vi "Sensors.vi"() -> ()   [LabVIEW 2020]
uses:
  <vilib>/Rock Robotics/SystemInterfaces/i2clib/i2c_bus.ctl
  <vilib>/Rock Robotics/SystemInterfaces/AI/FPGA_AIChannel.ctl
  <vilib>/Rock Robotics/WPI/ThirdParty/Phoenix-LabVIEW/Pigeon IMU/CTRE_PigeonIMU_TareType.ctl
  Team Code/Robot Global Data.vi
  <vilib>/Rock Robotics/WPI/ThirdParty/Phoenix-LabVIEW/Motor Controller/Get/CTRE_Phoenix_MotorController_IntegratedSensorData_TalonFX.vi
  <vilib>/Rock Robotics/WPI/ThirdParty/Phoenix-LabVIEW/Motor Controller/Get/CTRE_Phoenix_MotorController_GetSelectedSensorData.vi
  <vilib>/Rock Robotics/WPI/ThirdParty/Phoenix-LabVIEW/Pigeon IMU/CTRE_PigeonIMU_GetYPR.vi
  <vilib>/Rock Robotics/WPI/ThirdParty/Phoenix-LabVIEW/CANCoder/Get/CTRE_Phoenix_CANcoder_GetSensorData.vi
panel:
  out "error out":errorcluster
  in  "colorThreshold":dbl=300.0
  in  "I2C Bus":T1=enum."I2C MXP"
  in  "Blue Calibration":cluster{"R":dbl, "G":dbl, "B":dbl}={"R"=0.175926, "G"=0.433962, "B"=0.386792}
  in  "Red Calibration":cluster{"R":dbl, "G":dbl, "B":dbl}={"R"=0.462185, "G"=0.38843, "B"=0.15126}
  in  "Yellow Calibration":cluster{"R":dbl, "G":dbl, "B":dbl}={"R"=0.361, "G"=0.524, "B"=0.113}
  in  "Hysteresis":dbl=0.15 format="%#_13g"
  in  "Voltage Threshold":dbl=0.7 format="%#_13g"
  out "Color":u32(colorbox)
  out "Measured Color":cluster{"R":dbl, "G":dbl, "B":dbl}
  out "LoopTime (ms)":u32
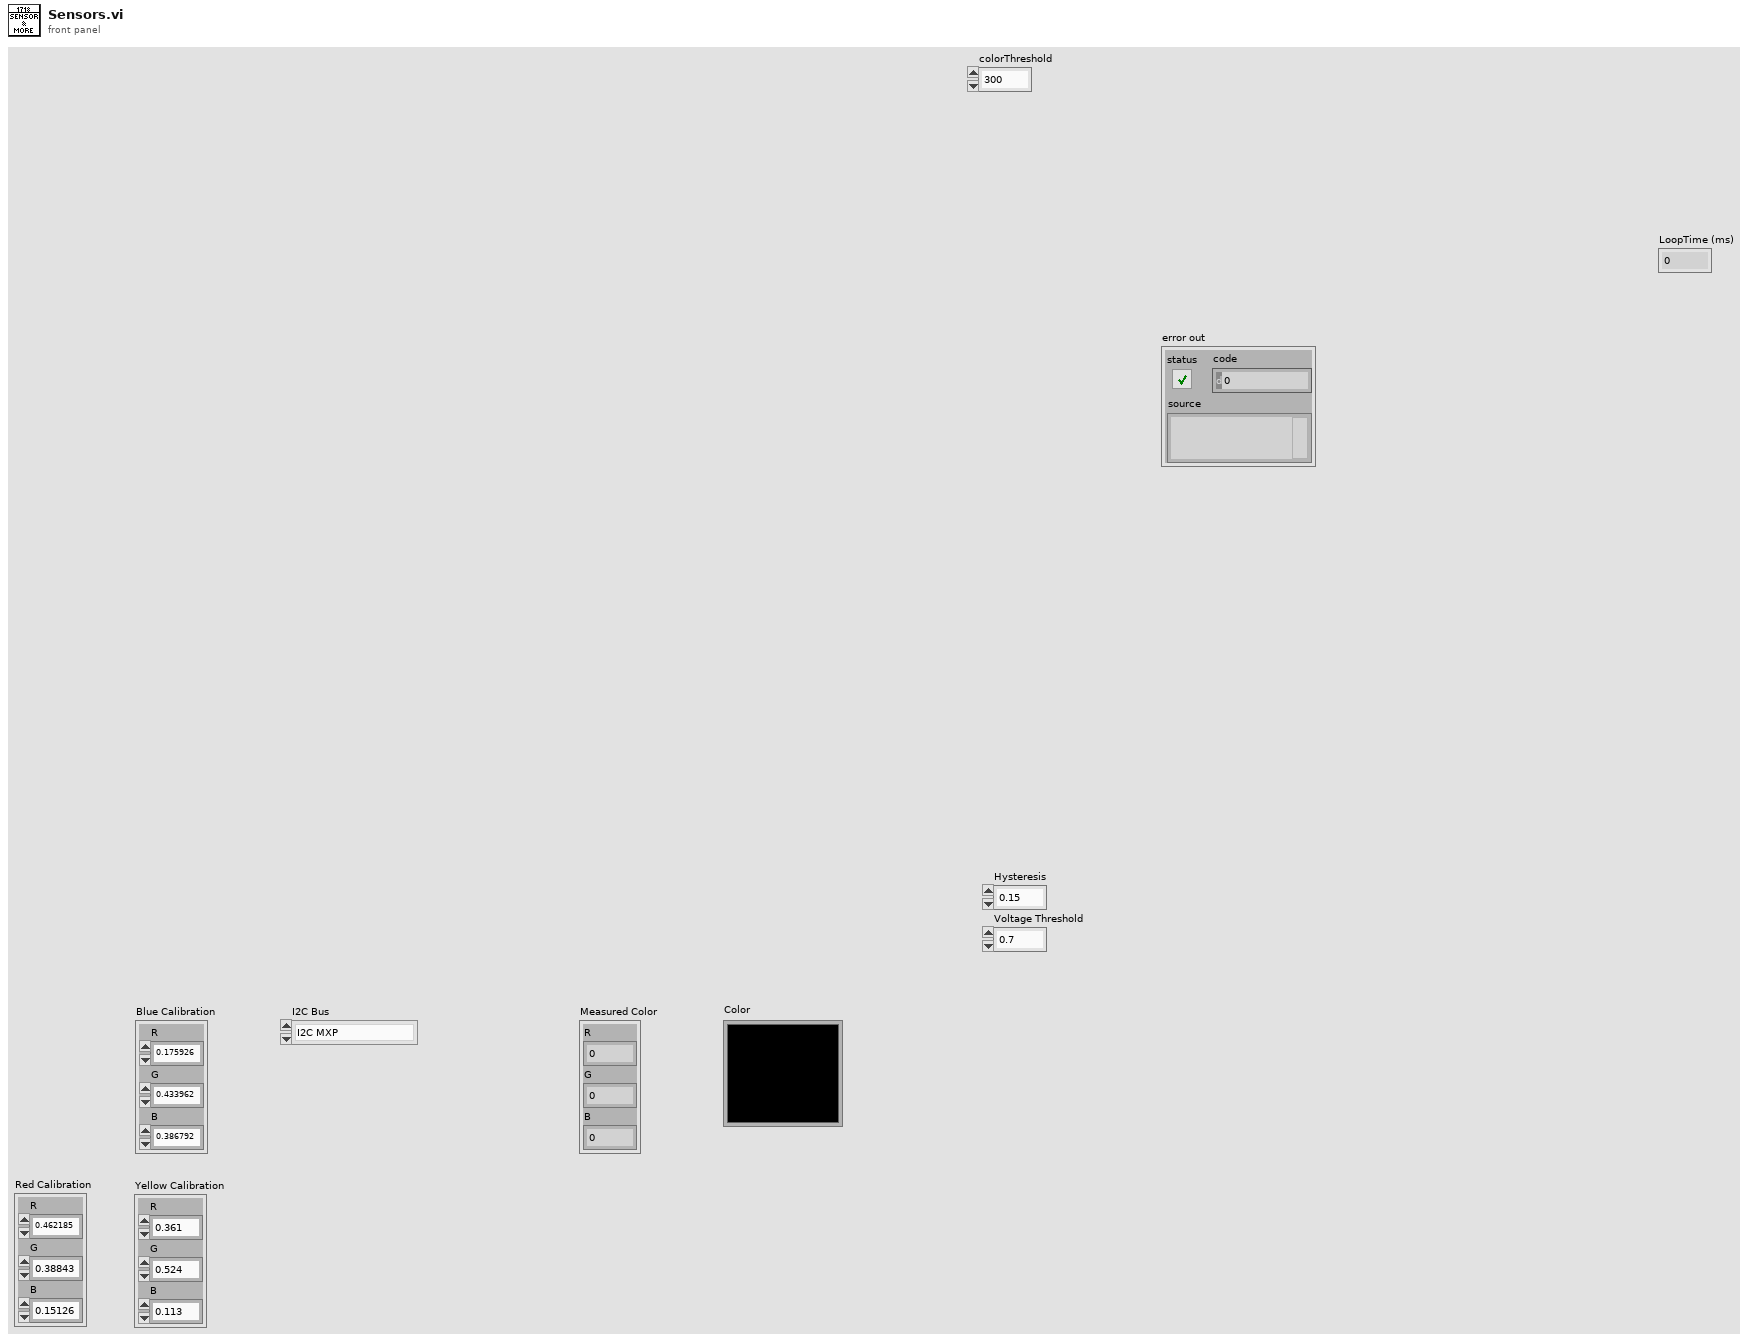
[diagram p1: front panel]
types:
  T1 = typedef "i2c_bus.ctl" = enum16{"I2C On-Board", "I2C MXP", "Invalid"}
  T2 = typedef "FPGA_AIChannel.ctl" = enum8{"AI 0", "AI 1", "AI 2", "AI 3", "AI MXP 0", "AI MXP 1", "AI MXP 2", "AI MXP 3", "Invalid"}
  T3 = typedef "PiConfig.ctl" = cluster{"swerveModules":cluster{"leftFront":T4, "rightFront":T4, "leftRear":T4, "rightRear":T4}, "offsets":cluster{"leftFrontAngleOffset":dbl, "leftRearAngleOffset":dbl, "rightFrontAngleOffset":dbl, "rightRearAngleOffset":dbl}, "limits":cluster{"maxVelocity":dbl, "maxOverdriveVelocity":dbl, "maxAcceleration":dbl, "maxPickupVelocity":dbl}, "speeds":cluster{"intakeSuckSpeed":dbl, "intakeSpitSpeed":dbl, "indexerSuckSpeed":dbl, "indexerSpitSpeed":dbl, "indexerShootSpeed":dbl, "indexerBumpBackSpeed":dbl, "shooterSpinupSpeed":dbl, "kickupSpinupSpeed":dbl, "shooterLowShootSpeed":dbl, "shooterHighShootSpeed":dbl}, "positions":cluster{"intakeStarting":dbl, "intakeStow":dbl, "intakeSuck":dbl, "armPounce":dbl, "armStow":dbl, "armUp":dbl, "winchPounce":dbl, "winchOut":dbl, "winchStow":dbl, "intakeSpit":dbl, "winchBarEngage":dbl, "winchBottomClimb":dbl, "hoodHighShoot":dbl, "armAirOut":dbl, "armAirUp":dbl, "winchAirOut":dbl, "winchAirUp":dbl, "winchHighClimb":dbl, "winchTraversalClimb":dbl}, "inversions":cluster{"rightShooter":bool, "leftShooter":bool}}
  T4 = typedef "Swerve Module Parameters.ctl" = cluster{"driveCANID":dbl, "angleCANID":i32, "canCoderCANID":dbl, "moduleName":string, "driveMotorNeutralMode":T5, "driveCurrentLimitConfig":T6, "driveFeedbackDevice":T7, "driveInitialSensorPosition":dbl, "driveEnableVoltageComp":bool, "driveVoltageComp":dbl, "driveRampRate":dbl, "angleCurrentLimit":dbl, "angleSensorType":T8, "angleMotorType":T9, "angleConversionFactor":dbl, "anglePIDRamp":dbl, "angleVoltageComp":dbl, "angleIdleMode":T10, "cancoderConfig":T11, "angleInitialSensorPosition":dbl}
  T5 = typedef "CTRE_Phoenix_MotorControl_NeutralMode.ctl" = enum8{"EEPROMSetting", "Override to Coast", "Override to Brake"}
  T6 = typedef "CTRE_Phoenix_MotorControl_SupplyCurrentLimitConfiguration.ctl" = cluster{"Enable?":bool, "Current Limit":dbl, "Threshold Current":dbl, "Threshold Time":dbl}
  T7 = typedef "CTRE_Phoenix_MotorControl_FeedbackDevice_TalonFX.ctl" = i8
  T8 = typedef "Spark MAX Sensor Type.ctl" = enum16{"No Sensor", "Hall Sensor", "Encoder", "-Not Available-", "Analog", "Alternate Encoder"}
  T9 = typedef "Spark MAX Motor Type.ctl" = enum16{"Brushed", "Brushless"}
  T10 = typedef "Spark MAX Idle Mode.ctl" = enum16{"Coast", "Brake"}
  T11 = typedef "CTRE_Phoenix_CANcoder_Configurables.ctl" = cluster{"Sensor Initialization Strategy":T12, "Absolute Sensor Range":T13, "Velocity Measurement Period":T14, "Velocity Measurement Window":i32, "Magnet Offset (Degrees)":dbl, "Sensor Direction":bool, "Sensor Coefficient":dbl, "Unit String":string, "Sensor Time Base":T15}
  T12 = typedef "CTRE_Phoenix_CANcoder_SensorInitializationStrategy.ctl" = enum16{"Boot To Zero", "Boot To Absolute Position"}
  T13 = typedef "CTRE_Phoenix_CANcoder_AbsoluteSensorRange.ctl" = enum16{"Unsigned [0 to 360)", "Signed [-180 to +180)"}
  T14 = typedef "CTRE_Phoenix_MotorControl_VelocityMeasurementPeriod.ctl" = u16
  T15 = typedef "CTRE_Phoenix_CANcoder_SensorTimeBase.ctl" = enum16{"Per100Ms_Legacy", "PerSecond", "PerMinute"}
  T16 = typedef "Color Sensor V3 DevRef.ctl" = cluster{"I2CDevRef":T17}
  T17 = typedef "WPI_I2CDevRef.ctl" = cluster{"DevStatus":errorcluster, "Device Address":u8, "Handle":i32, "I2C Bus":T1}
  T18 = typedef "WPI_AnalogChannelDevRef.ctl" = cluster{"DevStatus":errorcluster, "Analog Channel":T2}
  T19 = typedef "CTRE_Phoenix_CANcoder_DeviceRef.ctl" = cluster{"DeviceStatus":errorcluster, "Device Number":u8, "Handle":u64, "UsageFrame":u32, "Library Path":path}
  T20 = typedef "WPI_MotorControlDeviceRef.ctl" = cluster{"DeviceStatus":errorcluster, "Type":T21, "PWM":cluster{"PWM Channel":T22, "DeadBand":T23}, "CAN":cluster{"Device Number":u8, "SetOutput VI Ref":variant, "GetOutput VI Ref":variant, "Enable VI Ref":variant, "Disable VI Ref":variant, "Data":variant}, "Invert":bool, "DIO PWM":cluster{"PWM \"Enable\" Channel":T22, "DIOChannel":T24, "PWM Rate":dbl}}
  T21 = typedef "WPI_MotorControlType.ctl" = enum16{"PWM", "CAN", "DIO PWM"}
  T22 = typedef "FPGA_DIOPWMChannel.ctl" = enum8{"PWM 0", "PWM 1", "PWM 2", "PWM 3", "PWM 4", "PWM 5", "PWM 6", "PWM 7", "PWM 8", "PWM 9", "PWM MXP 0", "PWM MXP 1", "PWM MXP 2", "PWM MXP 3", "PWM MXP 4", "PWM MXP 5", "PWM MXP 6", "PWM MXP 7", "PWM MXP 8", "PWM MXP 9", "Invalid"}
  T23 = typedef "WPI_PWMDeadband.ctl" = cluster{"Name":string, "maxPositivePwm":i32, "minPositivePwm":i32, "centerPwm":i32, "maxNegativePwm":i32, "minNegativePwm":i32, "angularRange":u16}
  T24 = typedef "FPGA_DIOChannel.ctl" = enum8{"DIO 0", "DIO 1", "DIO 2", "DIO 3", "DIO 4", "DIO 5", "DIO 6", "DIO 7", "DIO 8", "DIO 9", "DIO MXP 0", "DIO MXP 1", "DIO MXP 2", "DIO MXP 3", "DIO MXP 4", "DIO MXP 5", "DIO MXP 6", "DIO MXP 7", "DIO MXP 8", "DIO MXP 9", "DIO MXP 10", "DIO MXP 11", "DIO MXP 12", "DIO MXP 13", "DIO MXP 14", "DIO MXP 15", "SPI Port CS1", "SPI Port CS2", "SPI Port CS3", "SPI Port MISO", "SPI Port MOSI", "Invalid"}
  T25 = typedef "CTRE_PigeonIMU_DeviceRef.ctl" = cluster{"DeviceStatus":errorcluster, "Device Number":u8, "Type":T26, "Device ID":u32, "Handle":u64, "UsageFrame":u32, "Library Path":path}
  T26 = typedef "CTRE_PigeonIMU_ConnectionType.ctl" = u32
  T27 = typedef "WPI_DriverStationAllianceInfo.ctl" = enum16{"Red", "Blue", "Invalid"}
  T28 = typedef "CTRE_PigeonIMU_TareType.ctl" = u8
  T29 = cluster{"offsetAngle H":dbl, "offsetAngle V":dbl, "area":dbl, "skew":dbl}
  T30 = cluster{"rightFrontDrivePositionTicks":dbl, "leftFrontDrivePositionTicks":dbl, "leftRearDrivePositionTicks":dbl, "rightRearDrivePositionTicks":dbl}
  T31 = cluster{"leftFrontDriveVelocityTicksPer100ms":dbl, "leftRearDriveVelocityTicksPer100ms":dbl, "rightFrontDriveVelocityTicksPer100ms":dbl, "rightRearDriveVelocityTicksper100ms":dbl}
  T32 = typedef "Absolute Angle TypeDef.ctl" = cluster{"leftFrontAbsoluteAngle":dbl, "leftRearAbsoluteAngle":dbl, "rightFrontAbsoluteAngle":dbl, "rightRearAbsoluteAngle":dbl}
  T33 = typedef "Cargo Sensors.ctl" = cluster{"ballPresent0":bool, "ballPresent1":bool, "ballPresent2":bool, "colorIsCorrect":bool, "ballPresent3":bool}
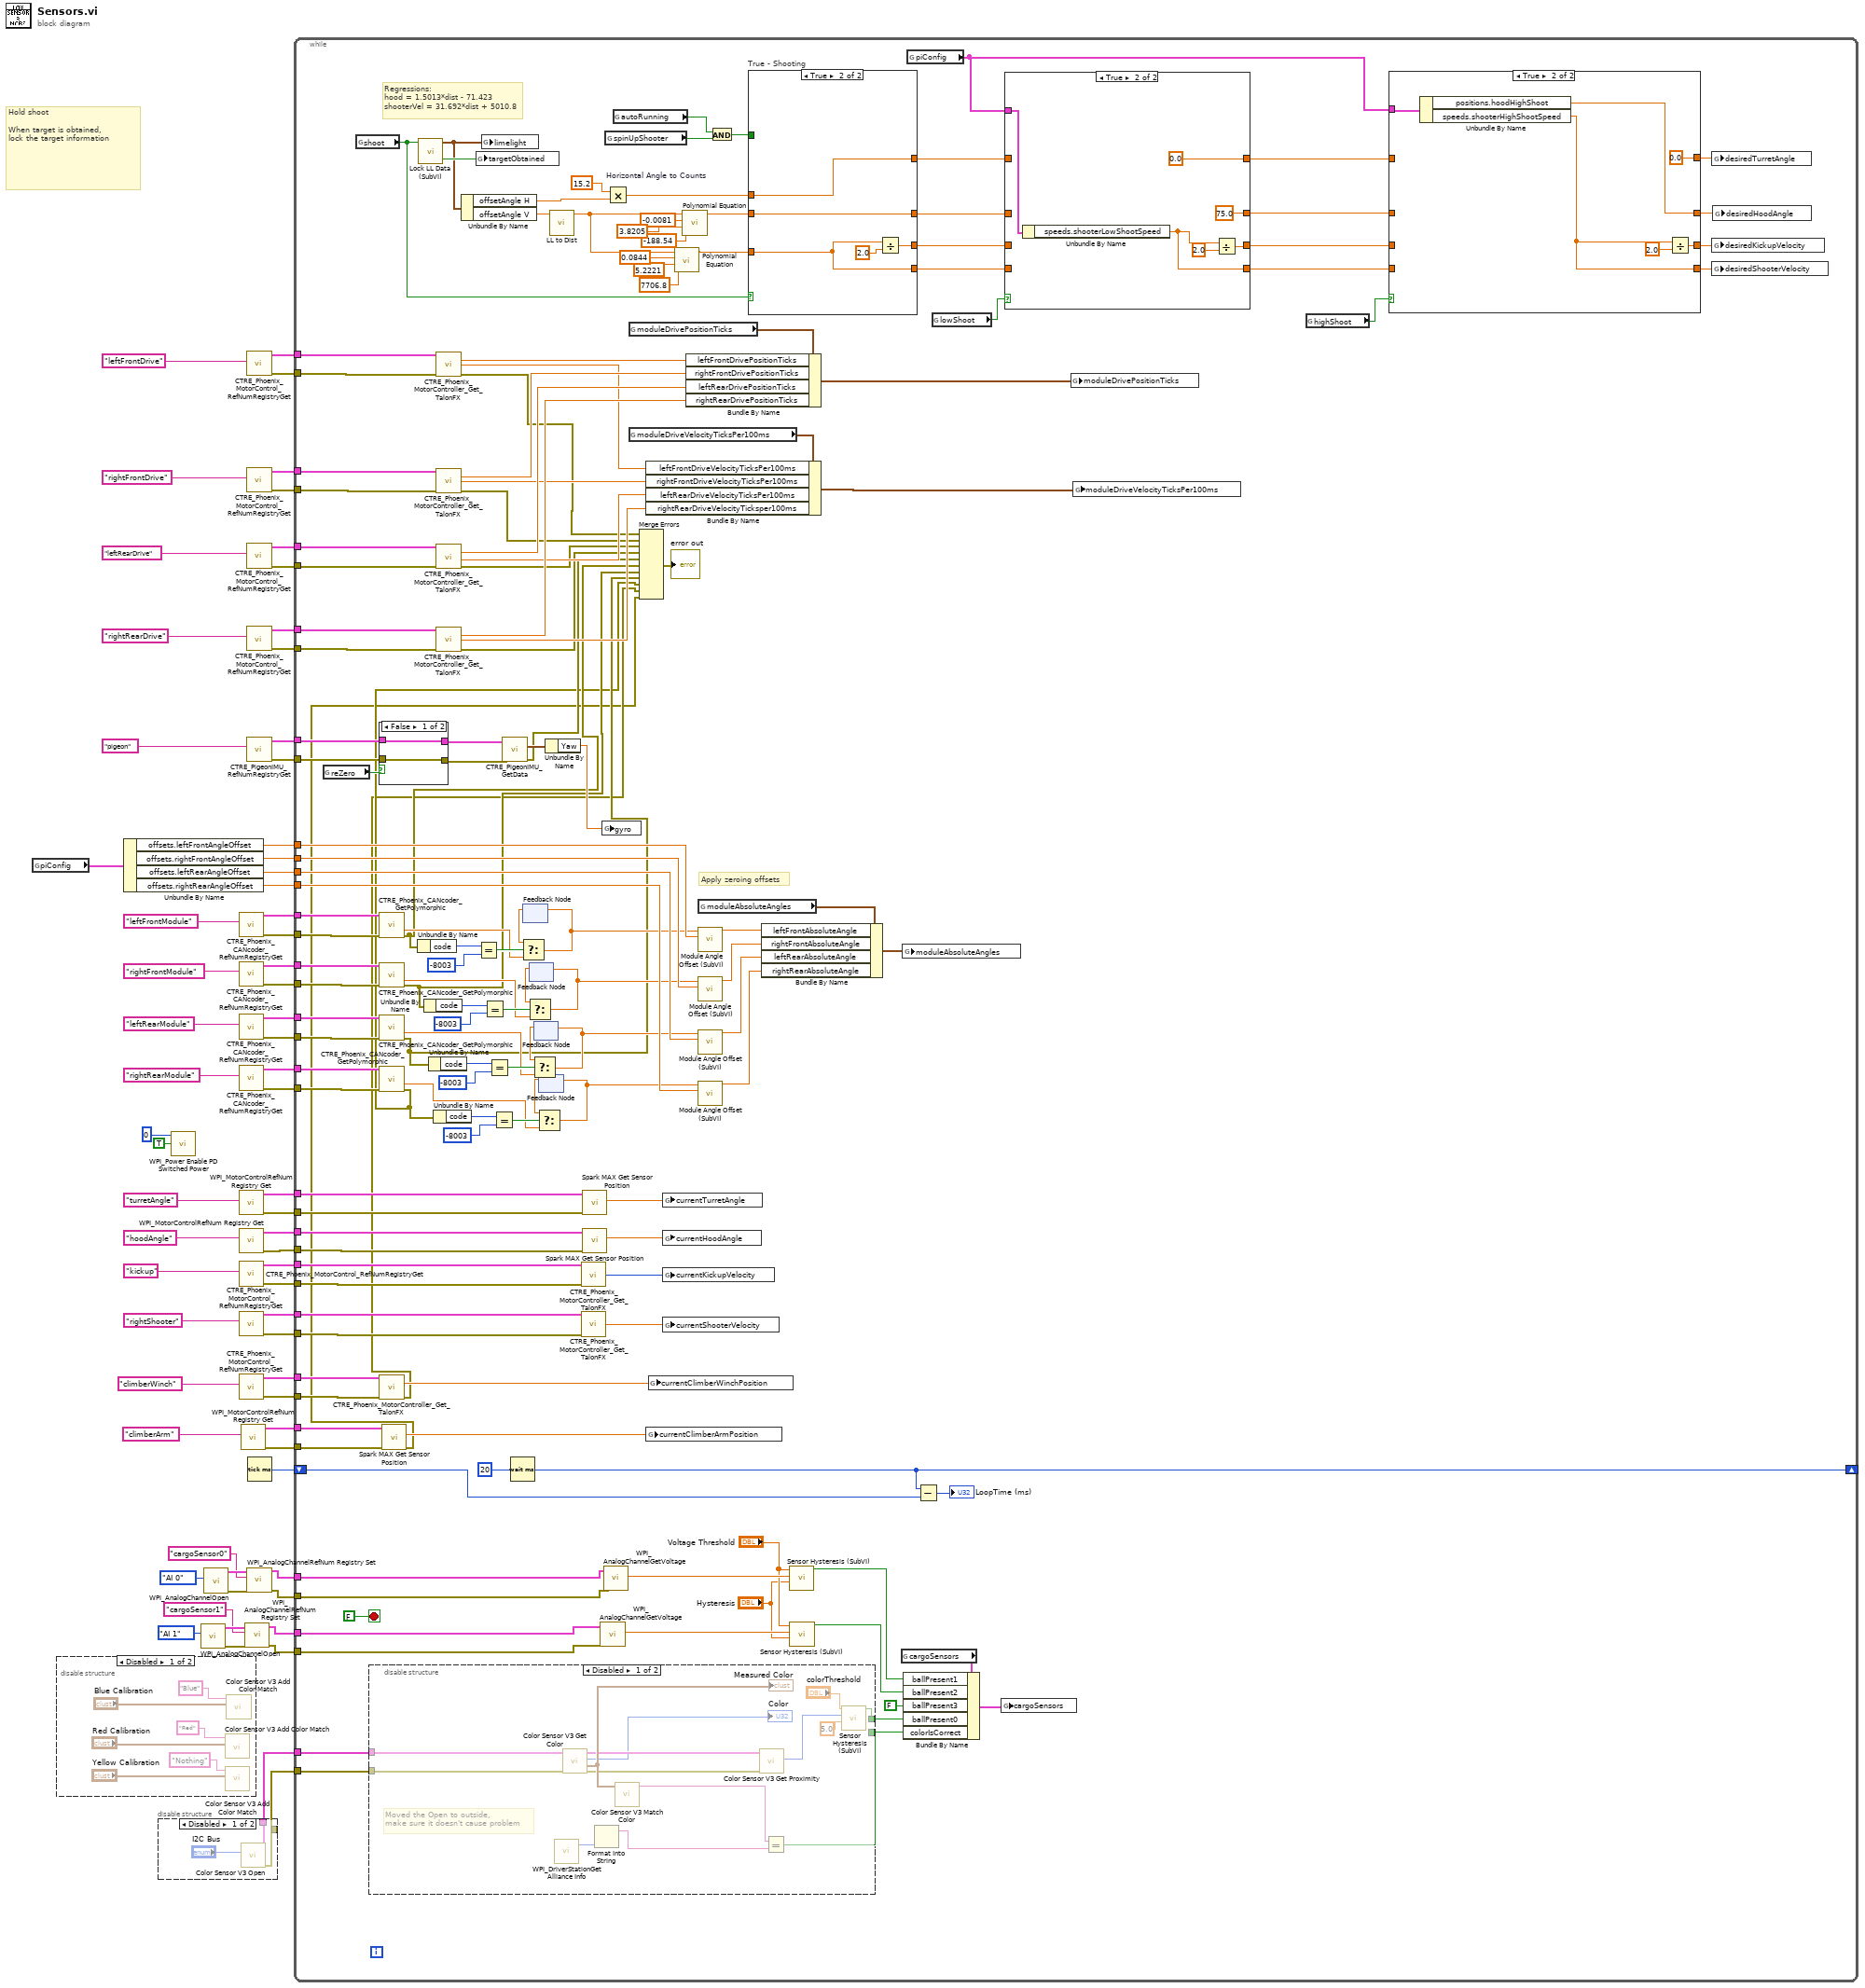
[diagram p0: block diagram]
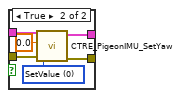
[diagram p4: hidden frame]
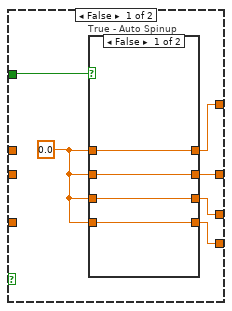
[diagram p8: hidden frame]
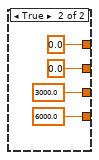
[diagram p9: hidden frame]
diagram:
  # "Hold shoot\n\nWhen target is obtained,\nlock the target information"
  n1 = global read "Robot Global Data.vi" "piConfig"() -> (w55:T3)
  n2 = disable-structure shown="Disabled" {
    frame Disabled {
      n3 = call <vilib>:"Color Sensor V3 Add Color Match.vi"("Color"="Red Calibration", "Name"="Red") -> ()  [unwired: 10 in]
      n4 = call <vilib>:"Color Sensor V3 Add Color Match.vi"("Color"="Yellow Calibration", "Name"="Nothing") -> ()  [unwired: 10 in]
      n5 = call <vilib>:"Color Sensor V3 Add Color Match.vi"("Color"="Blue Calibration", "Name"="Blue") -> ()  [unwired: 10 in]
    }
    frame Enabled {
    }
  }
  n6 = Unbundle By Name(w55) -> ("offsets.leftFrontAngleOffset"=w49:dbl, "offsets.rightFrontAngleOffset"=w48:dbl, "offsets.leftRearAngleOffset"=w47:dbl, "offsets.rightRearAngleOffset"=w46:dbl)
  n7 = disable-structure shown="Disabled" {
    disable-tunnel: [w76 _] -> w18
    disable-tunnel: [w75 _] -> w17
    frame Disabled {
      n8 = call <vilib>:"Color Sensor V3 Open.vi"("I2C Bus"="I2C Bus") -> ("error out"=w76:errorcluster, "ColorSensorDevRef"=w75:T16)  [unwired: 9 in]
    }
    frame Enabled {
    }
  }
  n9 = call <vilib>:"WPI_Power Enable PD Switched Power.vi"("Power Distribution (def)"=u8 0, "Switch Channel Value"=TRUE) -> ()  [unwired: 12 in, 2 out]
  n10 = call <vilib>:"WPI_AnalogChannelOpen.vi"("Analog Channel"=FPGA_AIChannel."AI 1") -> ("error out"=w16:errorcluster, "AIDeviceRef"=w15:T18)  [unwired: 9 in]
  n11 = call <vilib>:"WPI_AnalogChannelOpen.vi"("Analog Channel"=FPGA_AIChannel."AI 0") -> ("error out"=w13:errorcluster, "AIDeviceRef"=w14:T18)  [unwired: 9 in]
  n12 = call <vilib>:"CTRE_Phoenix_CANcoder_RefNumRegistryGet.vi"("refnum name"="leftFrontModule") -> ("error out"=w44:errorcluster, "CTRE_CANcoder_DeviceRef"=w45:T19)  [unwired: 9 in]
  n13 = call <vilib>:"CTRE_Phoenix_CANcoder_RefNumRegistryGet.vi"("refnum name"="rightFrontModule") -> ("error out"=w42:errorcluster, "CTRE_CANcoder_DeviceRef"=w43:T19)  [unwired: 9 in]
  n14 = call <vilib>:"CTRE_Phoenix_CANcoder_RefNumRegistryGet.vi"("refnum name"="leftRearModule") -> ("error out"=w40:errorcluster, "CTRE_CANcoder_DeviceRef"=w41:T19)  [unwired: 9 in]
  n15 = call <vilib>:"CTRE_Phoenix_CANcoder_RefNumRegistryGet.vi"("refnum name"="rightRearModule") -> ("error out"=w38:errorcluster, "CTRE_CANcoder_DeviceRef"=w39:T19)  [unwired: 9 in]
  n16 = call <vilib>:"WPI_MotorControlRefNum Registry Get.vi"("refnum name"="turretAngle") -> ("error out"=w32:errorcluster, "MotorControlDevRef"=w33:T20)  [unwired: 9 in]
  n17 = call <vilib>:"WPI_MotorControlRefNum Registry Get.vi"("refnum name"="hoodAngle") -> ("error out"=w31:errorcluster, "MotorControlDevRef"=w30:T20)  [unwired: 9 in]
  n18 = call <vilib>:"CTRE_Phoenix_MotorControl_RefNumRegistryGet.vi"("refnum name"="kickup") -> ("error out"=w25:errorcluster, "PhoenixMotorControlDevRef"=w26:T20)  [unwired: 9 in]
  n19 = call <vilib>:"CTRE_Phoenix_MotorControl_RefNumRegistryGet.vi"("refnum name"="rightShooter") -> ("error out"=w23:errorcluster, "PhoenixMotorControlDevRef"=w24:T20)  [unwired: 9 in]
  n20 = call <vilib>:"CTRE_Phoenix_MotorControl_RefNumRegistryGet.vi"("refnum name"="climberWinch") -> ("error out"=w8:errorcluster, "PhoenixMotorControlDevRef"=w7:T20)  [unwired: 9 in]
  n21 = call <vilib>:"WPI_MotorControlRefNum Registry Get.vi"("refnum name"="climberArm") -> ("error out"=w5:errorcluster, "MotorControlDevRef"=w4:T20)  [unwired: 9 in]
  n22 = call <vilib>:"WPI_AnalogChannelRefNum Registry Set.vi"("error in (no error)"=w16, "refnum name"="cargoSensor1", "AIDeviceRef"=w15) -> ("error out"=w22:errorcluster, "AIDeviceRef"=w21:T18)  [unwired: 7 in]
  n23 = call <vilib>:"CTRE_Phoenix_MotorControl_RefNumRegistryGet.vi"("refnum name"="leftFrontDrive") -> ("error out"=w62:errorcluster, "PhoenixMotorControlDevRef"=w63:T20)  [unwired: 9 in]
  n24 = call <vilib>:"CTRE_Phoenix_MotorControl_RefNumRegistryGet.vi"("refnum name"="rightFrontDrive") -> ("error out"=w60:errorcluster, "PhoenixMotorControlDevRef"=w61:T20)  [unwired: 9 in]
  n25 = call <vilib>:"CTRE_Phoenix_MotorControl_RefNumRegistryGet.vi"("refnum name"="leftRearDrive") -> ("error out"=w56:errorcluster, "PhoenixMotorControlDevRef"=w57:T20)  [unwired: 9 in]
  n26 = call <vilib>:"CTRE_Phoenix_MotorControl_RefNumRegistryGet.vi"("refnum name"="rightRearDrive") -> ("error out"=w58:errorcluster, "PhoenixMotorControlDevRef"=w59:T20)  [unwired: 9 in]
  n27 = call <vilib>:"CTRE_PigeonIMU_RefNumRegistryGet.vi"("refnum name"="pigeon") -> ("error out"=w36:errorcluster, "PigeonIMUDevRef"=w37:T25)  [unwired: 9 in]
  n28 = call <vilib>:"WPI_AnalogChannelRefNum Registry Set.vi"("error in (no error)"=w13, "refnum name"="cargoSensor0", "AIDeviceRef"=w14) -> ("error out"=w20:errorcluster, "AIDeviceRef"=w19:T18)  [unwired: 7 in]
  n29 = Tick Count (ms)() -> (millisecond timer value=w35:u32)
  n30 = while {
    tunnel: w63 -> [w231]
    tunnel: w62 -> [w230]
    tunnel: w61 -> [w229]
    tunnel: w60 -> [w228]
    tunnel: w59 -> [w227]
    tunnel: w58 -> [w226]
    tunnel: w57 -> [w225]
    tunnel: w56 -> [w224]
    tunnel: w49 -> [w222]
    tunnel: w48 -> [w221]
    tunnel: w47 -> [w220]
    tunnel: w46 -> [w219]
    tunnel: w45 -> [w218]
    tunnel: w44 -> [w217]
    tunnel: w43 -> [w216]
    tunnel: w42 -> [w215]
    tunnel: w41 -> [w214]
    tunnel: w40 -> [w213]
    tunnel: w39 -> [w212]
    tunnel: w38 -> [w211]
    tunnel: w37 -> [w103]
    tunnel: w36 -> [w102]
    shift-right: [w189] -> _
    shift-left: w35 -> [w190]
    tunnel: w33 -> [w187]
    tunnel: w32 -> [w188]
    tunnel: w30 -> [w186]
    tunnel: w31 -> [w185]
    tunnel: w26 -> [w182]
    tunnel: w25 -> [w181]
    tunnel: w24 -> [w180]
    tunnel: w23 -> [w179]
    tunnel: w22 -> [w173]
    tunnel: w21 -> [w172]
    tunnel: w20 -> [w171]
    tunnel: w19 -> [w170]
    tunnel: w18 -> [w163]
    tunnel: w17 -> [w162]
    tunnel: w7 -> [w124]
    tunnel: w8 -> [w125]
    tunnel: w4 -> [w121]
    tunnel: w5 -> [w120]
    stop <- FALSE stop-if-true
    # "Regressions:\nhood = 1.5013*dist - 71.423\nshooterVel = 31.692*dist + 5010.8"
    # "Apply zeroing offsets"
    n31 = global read "Robot Global Data.vi" "reZero"() -> (w99:bool)
    n32 = global read "Robot Global Data.vi" "shoot"() -> (w156:bool)
    n33 = disable-structure shown="Disabled" {
      disable-tunnel: [w273 _] -> w167
      disable-tunnel: [w272 _] -> w164
      disable-tunnel: w163 -> [w271 _]
      disable-tunnel: w162 -> [w270 _]
      frame Disabled {
        # "Moved the Open to outside,\nmake sure it doesn't cause problem"
        n34 = call <vilib>:"WPI_DriverStationGet Alliance Info.vi"() -> ("Alliance"=w268:T27)  [unwired: 6 in, 5 out]
        n35 = call <vilib>:"Color Sensor V3 Get Color.vi"("error in (no error)"=w271, "ColorSensorDevRef"=w270) -> ("error out"=w264:errorcluster, "Normalized Color"=w266:cluster{"R":dbl, "G":dbl, "B":dbl}, "Color"=→"Color":u32, "ColorSensorDevRef out"=w265:T16)  [unwired: 6 in]
        "Measured Color" <- w266
        n36 = Format Into String(w268) -> (resulting string=w269:string)  [unwired: 3 in, 1 out]
        n37 = call <vilib>:"Color Sensor V3 Match Color.vi"("Measured Color"=w266) -> ("Matched Color Name"=w267:string)  [unwired: 8 in, 2 out]
        n38 = call <vilib>:"Color Sensor V3 Get Proximity.vi"("error in (no error)"=w264, "ColorSensorDevRef"=w265) -> ("Proximity"=w261:u16)  [unwired: 7 in, 2 out]
        n39 = Equal?(x=w267, y=w269) -> (x = y?=w273:bool)
        n40 = call "Sensor Hysteresis (SubVI).vi"("Hysteresis"=5.0, "Input"=w261, "Threshold"="colorThreshold") -> ("Above Threshold"=w272:bool)  [unwired: 8 in]
      }
      frame Enabled {
      }
    }
    n41 = case shown="False" w99 {
      tunnel: w103 -> [w233 w239]
      tunnel: w102 -> [w232 w238]
      tunnel: [w233 w237] -> w101
      tunnel: [w232 w236] -> w100
      frame False {
      }
      frame True {
        w234 = T28 0 items=["SetValue"=0, "AddOffset"=1, "MatchCompass"=2, "SetOffset"=255] ("TareType (SetValue)")
        n42 = call <vilib>:"CTRE_PigeonIMU_SetYaw.vi"("error in (no error)"=w238, "TareType (SetValue)"=w234, "Value"=0.0, "PigeonIMUDevRef"=w239) -> ("error out"=w236:errorcluster, "PigeonIMUDevRef"=w237:T25)  [unwired: 6 in]
      }
    }
    n43 = call-poly <vilib>:"CTRE_Phoenix_CANcoder_GetPolymorphic.vi"("CTRE_CANcoder_DeviceRef"=w218, "error in"=w217) -> ("Absolute Position"=w145:dbl, "error out"=w83:errorcluster)  [unwired: 9 in, 3 out]
    n44 = call-poly <vilib>:"CTRE_Phoenix_CANcoder_GetPolymorphic.vi"("CTRE_CANcoder_DeviceRef"=w216, "error in"=w215) -> ("Absolute Position"=w131:dbl, "error out"=w82:errorcluster)  [unwired: 9 in, 3 out]
    n45 = call-poly <vilib>:"CTRE_Phoenix_CANcoder_GetPolymorphic.vi"("CTRE_CANcoder_DeviceRef"=w214, "error in"=w213) -> ("Absolute Position"=w129:dbl, "error out"=w81:errorcluster)  [unwired: 9 in, 3 out]
    n46 = call-poly <vilib>:"CTRE_Phoenix_CANcoder_GetPolymorphic.vi"("CTRE_CANcoder_DeviceRef"=w212, "error in"=w211) -> ("Absolute Position"=w128:dbl, "error out"=w80:errorcluster)  [unwired: 9 in, 3 out]
    n47 = call-poly <vilib>:"CTRE_Phoenix_MotorController_Get_TalonFX.vi"("PhoenixMotorControlDevRef"=w124, "error in"=w125) -> ("Position"=w123:dbl, "error out"=w79:errorcluster)  [unwired: 9 in, 3 out]
    n48 = call <vilib>:"Spark MAX Get Sensor Position.vi"("error in (no error)"=w120, "MotorControlDevRef in"=w121) -> ("error out"=w78:errorcluster, "Sensor Position"=w122:dbl)  [unwired: 6 in, 2 out]
    n49 = Unbundle By Name(w83) -> ("code"=w149:i32)
    n50 = call "Lock LL Data (SubVI).vi"("shoot"=w156) -> ("Boolean"=w176:bool, "Output cluster"=w175:T29)  [unwired: 9 in]
    n51 = Unbundle By Name(w82) -> ("code"=w143:i32)
    n52 = Unbundle By Name(w81) -> ("code"=w139:i32)
    n53 = Unbundle By Name(w80) -> ("code"=w135:i32)
    n54 = call-poly <vilib>:"CTRE_Phoenix_MotorController_Get_TalonFX.vi"("PhoenixMotorControlDevRef"=w231, "error in"=w230) -> ("Position"=w200:dbl, "Velocity"=w192:dbl, "error out"=w88:errorcluster)  [unwired: 9 in, 2 out]
    n55 = call-poly <vilib>:"CTRE_Phoenix_MotorController_Get_TalonFX.vi"("PhoenixMotorControlDevRef"=w229, "error in"=w228) -> ("Position"=w199:dbl, "Velocity"=w193:dbl, "error out"=w87:errorcluster)  [unwired: 9 in, 2 out]
    n56 = call-poly <vilib>:"CTRE_Phoenix_MotorController_Get_TalonFX.vi"("PhoenixMotorControlDevRef"=w225, "error in"=w224) -> ("Position"=w198:dbl, "Velocity"=w195:dbl, "error out"=w86:errorcluster)  [unwired: 9 in, 2 out]
    n57 = call-poly <vilib>:"CTRE_Phoenix_MotorController_Get_TalonFX.vi"("PhoenixMotorControlDevRef"=w227, "error in"=w226) -> ("Position"=w197:dbl, "Velocity"=w194:dbl, "error out"=w85:errorcluster)  [unwired: 9 in, 2 out]
    n58 = Unbundle By Name(w175) -> ("offsetAngle H"=w151:dbl, "offsetAngle V"=w161:dbl)
    n59 = global write "Robot Global Data.vi" "targetObtained"(w176) -> ()
    n60 = Equal?(x=w149, y=-8003) -> (x = y?=w147:bool)
    n61 = global write "Robot Global Data.vi" "limelight"(w175) -> ()
    n62 = Equal?(x=w143, y=-8003) -> (x = y?=w141:bool)
    n63 = Equal?(x=w139, y=-8003) -> (x = y?=w137:bool)
    n64 = Equal?(x=w135, y=-8003) -> (x = y?=w133:bool)
    n65 = call-poly <vilib>:"CTRE_PigeonIMU_GetData.vi"("error in (no error)"=w100, "PigeonIMUDevRef"=w101) -> ("error out"=w84:errorcluster, "Yaw Pitch Roll"=w202:cluster{"Yaw":dbl, "Pitch":dbl, "Roll":dbl})  [unwired: 7 in, 1 out]
    n66 = Wait (ms)(milliseconds to wait=u32 20) -> (millisecond timer value=w189:u32)
    n67 = feedback #1() -> (w144:dbl)  [unwired: 1 in]
    n68 = Select(t=w144, s=w147, f=w145) -> (s? t:f=w146:dbl)
    n69 = feedback-in #1(w146) -> ()
    n70 = feedback #2() -> (w140:dbl)  [unwired: 1 in]
    n71 = Select(t=w140, s=w141, f=w131) -> (s? t:f=w130:dbl)
    n72 = feedback-in #2(w130) -> ()
    n73 = feedback #3() -> (w136:dbl)  [unwired: 1 in]
    n74 = Select(t=w136, s=w137, f=w129) -> (s? t:f=w127:dbl)
    n75 = feedback-in #3(w127) -> ()
    n76 = feedback #4() -> (w132:dbl)  [unwired: 1 in]
    n77 = Select(t=w132, s=w133, f=w128) -> (s? t:f=w126:dbl)
    n78 = feedback-in #4(w126) -> ()
    n79 = Unbundle By Name(w202) -> ("Yaw"=w104:dbl)
    n80 = call "LL to Dist.vi"("limelightV"=w161) -> ("distance"=w92:dbl)  [unwired: 10 in]
    n81 = call-poly <vilib>:"CTRE_Phoenix_MotorController_Get_TalonFX.vi"("PhoenixMotorControlDevRef"=w182, "error in"=w181) -> ("Velocity (Raw Sensor Units per 100 ms)"=w178:i32)  [unwired: 10 in, 3 out]
    n82 = call-poly <vilib>:"CTRE_Phoenix_MotorController_Get_TalonFX.vi"("PhoenixMotorControlDevRef"=w180, "error in"=w179) -> ("Velocity"=w177:dbl)  [unwired: 9 in, 4 out]
    n83 = call <vilib>:"Spark MAX Get Sensor Position.vi"("error in (no error)"=w188, "MotorControlDevRef in"=w187) -> ("Sensor Position"=w183:dbl)  [unwired: 6 in, 3 out]
    n84 = call <vilib>:"Spark MAX Get Sensor Position.vi"("error in (no error)"=w185, "MotorControlDevRef in"=w186) -> ("Sensor Position"=w184:dbl)  [unwired: 6 in, 3 out]
    n85 = call <vilib>:"WPI_AnalogChannelGetVoltage.vi"("error in (no error)"=w173, "AIDeviceRef"=w172) -> ("Voltage"=w159:dbl)  [unwired: 7 in, 2 out]
    n86 = global write "Robot Global Data.vi" "gyro"(w104) -> ()
    n87 = call <vilib>:"WPI_AnalogChannelGetVoltage.vi"("error in (no error)"=w171, "AIDeviceRef"=w170) -> ("Voltage"=w160:dbl)  [unwired: 7 in, 2 out]
    n88 = global read "Robot Global Data.vi" "spinUpShooter"() -> (w155:bool)
    n89 = Multiply "Horizontal Angle to Counts"(x=15.2 ("Counts/H Degree"), y=w151) -> (x*y=w174:dbl)
    n90 = global read "Robot Global Data.vi" "autoRunning"() -> (w154:bool)
    n91 = global read "Robot Global Data.vi" "moduleDrivePositionTicks"() -> (w201:T30)
    n92 = global read "Robot Global Data.vi" "moduleDriveVelocityTicksPer100ms"() -> (w196:T31)
    n93 = Merge Errors(w88, w87, w86, w85, w84, w83, w82, w81, w80, w79, w78) -> (→"error out":errorcluster)
    n94 = Bundle By Name(cluster=w196, "leftFrontDriveVelocityTicksPer100ms"=w192, "rightFrontDriveVelocityTicksPer100ms"=w193, "leftRearDriveVelocityTicksPer100ms"=w195, "rightRearDriveVelocityTicksper100ms"=w194) -> (w210:T31)
    n95 = global write "Robot Global Data.vi" "currentClimberArmPosition"(w122) -> ()
    n96 = global write "Robot Global Data.vi" "currentClimberWinchPosition"(w123) -> ()
    n97 = global write "Robot Global Data.vi" "currentTurretAngle"(w183) -> ()
    n98 = global write "Robot Global Data.vi" "currentHoodAngle"(w184) -> ()
    n99 = global write "Robot Global Data.vi" "currentKickupVelocity"(w178) -> ()
    n100 = global write "Robot Global Data.vi" "currentShooterVelocity"(w177) -> ()
    n101 = call "Polynomial Equation.vi"("Y-Int"=7706.8, "Slope"=5.2221, "X^2 Coeff."=0.0844, "X"=w92) -> ("Output"=w93:dbl)  [unwired: 7 in]
    n102 = call "Polynomial Equation.vi"("Y-Int"=-188.54, "Slope"=3.8205, "X^2 Coeff."=-0.0081, "X"=w92) -> ("Output"=w97:dbl)  [unwired: 7 in]
    n103 = Bundle By Name(cluster=w201, "leftFrontDrivePositionTicks"=w200, "rightFrontDrivePositionTicks"=w199, "leftRearDrivePositionTicks"=w198, "rightRearDrivePositionTicks"=w197) -> (w209:T30)
    n104 = global read "Robot Global Data.vi" "moduleAbsoluteAngles"() -> (w203:T32)
    n105 = call "Module Angle Offset (SubVI).vi"("angleOffset"=w222, "absoluteAngle"=w146) -> ("absoluteAngle"=w208:dbl)  [unwired: 9 in]
    n106 = call "Module Angle Offset (SubVI).vi"("angleOffset"=w221, "absoluteAngle"=w130) -> ("absoluteAngle"=w205:dbl)  [unwired: 9 in]
    n107 = call "Module Angle Offset (SubVI).vi"("angleOffset"=w220, "absoluteAngle"=w127) -> ("absoluteAngle"=w206:dbl)  [unwired: 9 in]
    n108 = call "Module Angle Offset (SubVI).vi"("angleOffset"=w219, "absoluteAngle"=w126) -> ("absoluteAngle"=w207:dbl)  [unwired: 9 in]
    n109 = And(x=w154, y=w155) -> (x .and. y?=w153:bool)
    n110 = case "True - Shooting" shown="True" w156 {
      tunnel: w174 -> [_ w292]
      tunnel: w97 -> [_ w291]
      tunnel: w93 -> [_ w288]
      tunnel: w153 -> [w279 _]
      tunnel: [w277 w292] -> w119
      tunnel: [w276 w291] -> w118
      tunnel: [w275 w290] -> w117
      tunnel: [w274 w288] -> w116
      frame False {
        w278 = 0.0 ("y")
        n111 = case "True - Auto Spinup" shown="False" w279 {
          tunnel: [w283 0.0 ("y")] -> w277
          tunnel: w278 -> [w283 _]
          tunnel: [w282 0.0 ("Output")] -> w276
          tunnel: w278 -> [w282 _]
          tunnel: [w281 3000.0 ("y")] -> w275
          tunnel: w278 -> [w281 _]
          tunnel: [w280 6000.0 ("Output")] -> w274
          tunnel: w278 -> [w280 _]
          frame False {
          }
          frame True {
          }
        }
      }
      frame True {
        n112 = Divide(x=w288, y=2.0) -> (x/y=w290:dbl)
      }
    }
    n113 = Bundle By Name(cluster=w203, "leftFrontAbsoluteAngle"=w208, "rightFrontAbsoluteAngle"=w205, "leftRearAbsoluteAngle"=w206, "rightRearAbsoluteAngle"=w207) -> (w204:T32)
    n114 = call "Sensor Hysteresis (SubVI).vi"("Hysteresis"="Hysteresis", "Input"=w160, "Threshold"="Voltage Threshold") -> ("Above Threshold"=w166:bool)  [unwired: 8 in]
    n115 = call "Sensor Hysteresis (SubVI).vi"("Hysteresis"="Hysteresis", "Input"=w159, "Threshold"="Voltage Threshold") -> ("Above Threshold"=w165:bool)  [unwired: 8 in]
    n116 = global read "Robot Global Data.vi" "cargoSensors"() -> (w169:T33)
    n117 = global write "Robot Global Data.vi" "moduleAbsoluteAngles"(w204) -> ()
    n118 = Bundle By Name(cluster=w169, "ballPresent1"=w166, "ballPresent2"=w165, "ballPresent3"=FALSE, "ballPresent0"=w164, "colorIsCorrect"=w167) -> (w168:T33)
    n119 = global read "Robot Global Data.vi" "piConfig"() -> (w105:T3)
    n120 = Subtract(x=w189, y=w190) -> (x-y=→"LoopTime (ms)":u32)
    n121 = global read "Robot Global Data.vi" "lowShoot"() -> (w115:bool)
    n122 = global write "Robot Global Data.vi" "cargoSensors"(w168) -> ()
    n123 = case shown="True" w115 {
      tunnel: w119 -> [w253 _]
      tunnel: w118 -> [w252 _]
      tunnel: w117 -> [w251 _]
      tunnel: w116 -> [w250 _]
      tunnel: [w253 0.0 ("y")] -> w113
      tunnel: [w252 75.0 ("Output")] -> w112
      tunnel: [w251 w256] -> w111
      tunnel: [w250 w254] -> w110
      tunnel: w105 -> [_ w257]
      frame False {
      }
      frame True {
        n124 = Unbundle By Name(w257) -> ("speeds.shooterLowShootSpeed"=w254:dbl)
        n125 = Divide(x=w254, y=2.0) -> (x/y=w256:dbl)
      }
    }
    n126 = global write "Robot Global Data.vi" "moduleDrivePositionTicks"(w209) -> ()
    n127 = global write "Robot Global Data.vi" "moduleDriveVelocityTicksPer100ms"(w210) -> ()
    n128 = global read "Robot Global Data.vi" "highShoot"() -> (w114:bool)
    n129 = case shown="True" w114 {
      tunnel: [w243 0.0 ("y")] -> w109
      tunnel: w113 -> [w243 _]
      tunnel: [w242 w247] -> w108
      tunnel: w112 -> [w242 _]
      tunnel: w111 -> [w241 _]
      tunnel: w110 -> [w240 _]
      tunnel: [w241 w246] -> w107
      tunnel: [w240 w245] -> w106
      tunnel: w105 -> [_ w248]
      frame False {
      }
      frame True {
        n130 = Unbundle By Name(w248) -> ("positions.hoodHighShoot"=w247:dbl, "speeds.shooterHighShootSpeed"=w245:dbl)
        n131 = Divide(x=w245, y=2.0) -> (x/y=w246:dbl)
      }
    }
    n132 = global write "Robot Global Data.vi" "desiredTurretAngle"(w109) -> ()
    n133 = global write "Robot Global Data.vi" "desiredKickupVelocity"(w107) -> ()
    n134 = global write "Robot Global Data.vi" "desiredShooterVelocity"(w106) -> ()
    n135 = global write "Robot Global Data.vi" "desiredHoodAngle"(w108) -> ()
  }
